vi "Land.vi"(10 "NavData Port":refnum<k16>, 11 "AT Command Port":refnum<k16>) -> (2 "NavData Port":refnum<k16>, 3 "AT Command Port":refnum<k16>)   [LabVIEW 2011]
panel:
  in  "stop":bool
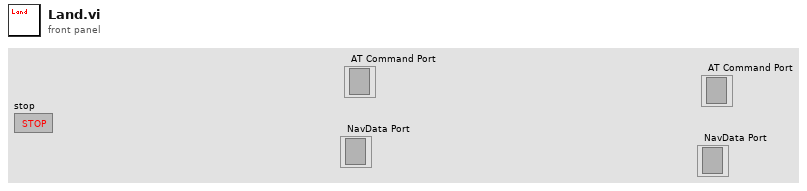
[diagram p1: front panel]
types:
  T1 = cluster{"Drone Status Bits":cluster{"Flying?":bool, "Video Enabled?":bool, "Vision Enabled?":bool, "Angular Speed Control?":bool, "Altitude Control?":bool, "Start button?":bool, "Control Command Recieved?":bool, "Trim Command Recieved?":bool, "Trim Running?":bool, "Trim Succeeded?":bool, "Navdata Demo Mode?":bool, "Navdata Bootstrap Mode?":bool, "Motors Com Down?":bool, "Unknown":bool, "Gyrometer Problem?":bool, "Battery Voltage Too Low?":bool, "Battery Voltage Too High?":bool, "Timer Elapsed?":bool, "Power Too Low?":bool, "Angles Out Of Range?":bool, "Too Much Wind?":bool, "Ultrasound Deaf?":bool, "Cutout Detected?":bool, "PIC Version Number OK?":bool, "ATCodec Thread On?":bool, "Navdata Thread On?":bool, "Video Thread On?":bool, "Acquisition Thread On?":bool, "Control Watchdog Delay?":bool, "ADC Watchdog Delay?":bool, "Communications Problem?":bool, "Emergency?":bool}, "Header":u32, "Sequence Number":u32, "Vision Defined?":bool, "Blocks":cluster{"Size":u16, "Data":u8[], "ID":enum16{"NAVDATA_DEMO", "NAVDATA_TIME", "NAVDATA_RAW_MEASURES", "NAVDATA_PHYS_MEASURES", "NAVDATA_GYROS_OFFSETS", "NAVDATA_EULER_ANGLES", "NAVDATA_REFERENCES", "NAVDATA_TRIMS", "NAVDATA_RC_REFERENCES", "NAVDATA_PWM", "NAVDATA_ALTITUDE", "NAVDATA_VISION_RAW", "NAVDATA_VISION_OF", "NAVDATA_VISION", "NAVDATA_VISION_PERF", "NAVDATA_TRACKERS_SEND", "NAVDATA_VISION_DETECT", "NAVDATA_WATCHDOG", "NAVDATA_ADC_DATA_FRAME", "NAVDATA_VIDEO_STREAM", "NAVDATA_GAMES"}}[]}
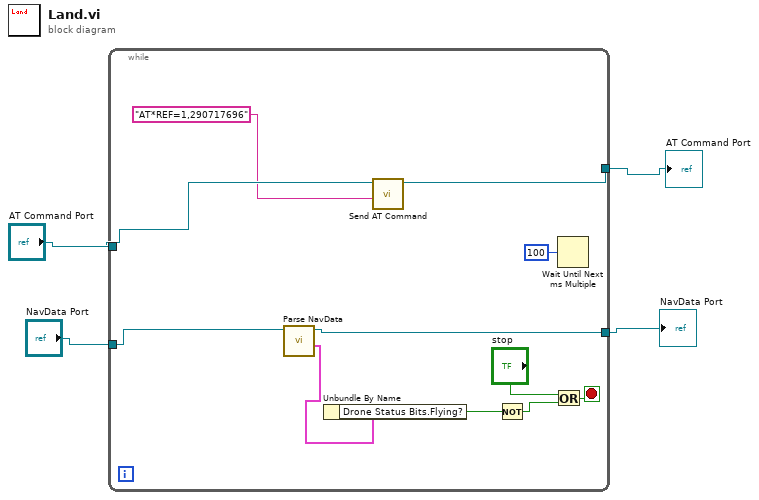
[diagram p0: block diagram]
diagram:
  n1 = while {
    tunnel: "NavData Port" -> [w9]
    tunnel: [w8] -> w1
    tunnel: "AT Command Port" -> [w12]
    tunnel: [w11] -> w4
    stop <- w14 stop-if-true
    n2 = call "Parse NavData.vi"("NavData Port"=w9) -> ("NavData"=w7:T1, "NavData Port"=w8:refnum<k16>)  [unwired: 9 in]
    n3 = Unbundle By Name(w7) -> ("Drone Status Bits.Flying?"=w6:bool)
    n4 = call "Send AT Command.vi"("AT Command"="AT*REF=1,290717696", "AT Command Port"=w12) -> ("AT Command Port"=w11:refnum<k16>)  [unwired: 9 in]
    n5 = Not(x=w6) -> (.not. x?=w5:bool)
    n6 = Or(x="stop", y=w5) -> (x .or. y?=w14:bool)
    n7 = Wait Until Next ms Multiple(millisecond multiple=u32 100) -> ()  [unwired: 1 out]
  }
  "AT Command Port" <- w4
  "NavData Port" <- w1
